vi "init.vi"(8 "error in":errorcluster, 10 "TBM module configuration in":refnum<class "TBM module configuration.lvclass">, 11 "fixed channel runtime in":refnum<class "GPIC ScaleAndLimit runtime.lvclass">) -> (0 "error out":errorcluster, 1 "data allocations":T1, 2 "execution settings":T4, 3 "fixed channel runtime out":refnum<class "GPIC ScaleAndLimit runtime.lvclass">)   [LabVIEW 2015, in "GPIC ScaleAndLimit runtime.lvclass"]
doc: "Provides an interface for initializing a module at runtime. While this interface performs no operations, a child should provide an override which may open any necessary references or sessions, allocate necessary memory, and perform any final configuration validataion before providing the full configuration <b>execution data</b> to the calling process."
uses:
  GPIC ScaleAndLimit runtime.lvclass
  <vilib>/NI/Tag Bus Module Framework/module configuration/TBM module configuration.lvclass
  <vilib>/NI/Tag Bus Module Framework/runtime/execution settings.ctl
  <vilib>/NI/Tag Bus Module Framework/channel/data tables.ctl
  <vilib>/NI/Tag Bus/dictionary/data dictionary.lvclass
  <vilib>/NI/Tag Bus/dictionary table pair.ctl
  <vilib>/NI/Tag Bus/table/data table.ctl
  <vilib>/NI/Tag Bus Module Framework/FPGA manager/methods.ctl
  <vilib>/userdefined/High Color/nirio_resource_hc.ctl
  Interface/FPGAInterface.ctl
  configuration/GPIC ScaleAndLimit configuration.lvclass
  Interface/Configuration.ctl
  GPIC ScaleAndLimit runtime.lvclass/GPIC ScaleAndLimit runtime.ctl
  <vilib>/NI/DCAF/Tag Editor Core/control module/runtime/control module runtime.lvclass
  <vilib>/NI/Tag Bus Module Framework/FPGA manager/FPGA manager.lvlib
  Interface/ScaleAndLimitInterface.lvlib
  <vilib>/NI/Tag Bus Module Framework/runtime/TBM module execution interface.lvclass
  <vilib>/NI/Tag Bus Module Framework/channel/TBM channel.lvclass
  <vilib>/NI/Tag Bus/tag bus.lvlib
  <vilib>/NI/Tag Bus/table/data table.lvlib
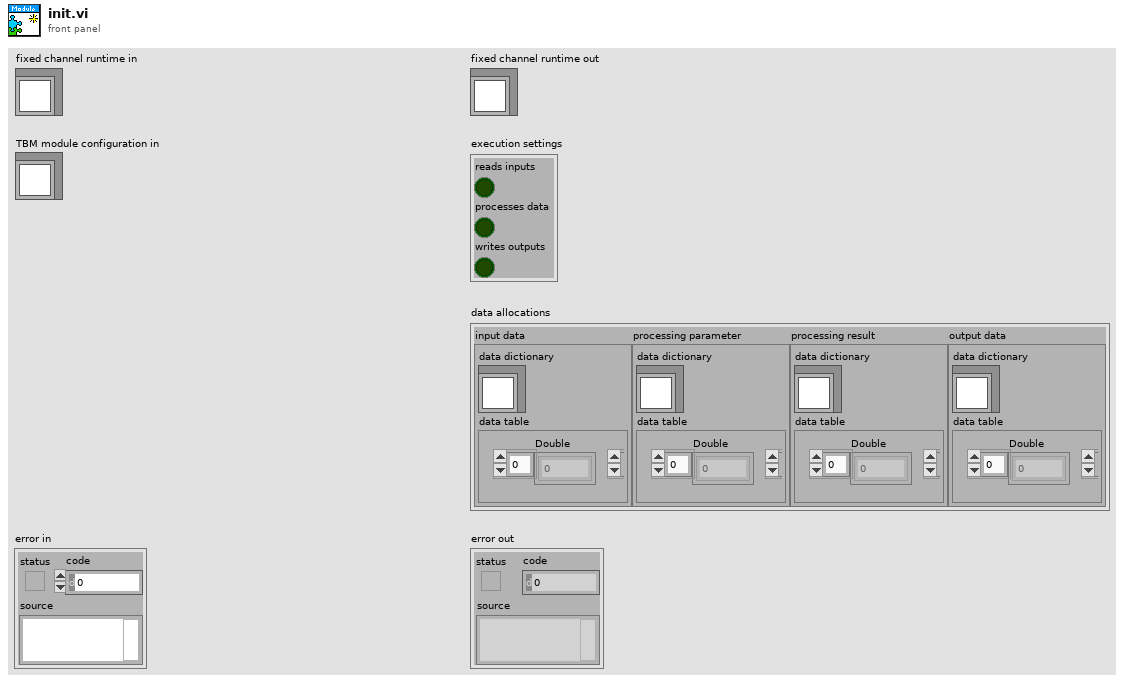
[diagram p1: front panel]
types:
  T1 = typedef "TBM channel.lvclass/data tables.ctl" = cluster{"input data":T2, "processing parameter":T2, "processing result":T2, "output data":T2}
  T2 = typedef "tag bus.lvlib/dictionary table pair.ctl" = cluster{"data dictionary":refnum<class "data dictionary.lvclass">, "data table":T3}
  T3 = typedef "tag bus.lvlib/data table.lvlib/data table.ctl" = cluster{"Double":dbl[], "Single":sgl[], "I64":i64[], "I32":i32[], "I16":i16[], "I8":i8[], "U64":u64[], "U32":u32[], "U16":u16[], "U8":u8[], "Boolean":bool[], "String":string[], "Array of Double":cluster{"DBL Array":dbl[]}[], "Array of Single":cluster{"SGL Array":sgl[]}[], "Array of I64":cluster{"I64 Array":i64[]}[], "Array of I32":cluster{"I32 Array":i32[]}[], "Array of I16":cluster{"I16 Array":i16[]}[], "Array of I8":cluster{"I8 Array":i8[]}[], "Array of U64":cluster{"U64 Array":u64[]}[], "Array of U32":cluster{"U32 Array":u32[]}[], "Array of U16":cluster{"U16 Array":u16[]}[], "Array of U8":cluster{"U8 Array":u8[]}[], "Array of Boolean":cluster{"Boolean Array":bool[]}[], "Array of String":cluster{"String Array":string[]}[]}
  T4 = typedef "TBM module execution interface.lvclass/execution settings.ctl" = cluster{"reads inputs":bool, "processes data":bool, "writes outputs":bool}
  T5 = typedef "ScaleAndLimitInterface.lvlib/Configuration.ctl" = cluster{"Name":string, "M":dbl, "B":i16, "HighLimit":dbl, "LowLimit":dbl, "LimitsEnabled":bool}
  T6 = typedef "ScaleAndLimitInterface.lvlib/FPGAInterface.ctl" = refnum<k20>
  T7 = typedef "nirio_resource_hc.ctl" = tag
  T8 = typedef "FPGA manager.lvlib/methods.ctl" = enum16{"initialize bitfile", "cache bitfile", "locate bitfile", "close bitfile", "clear manager"}
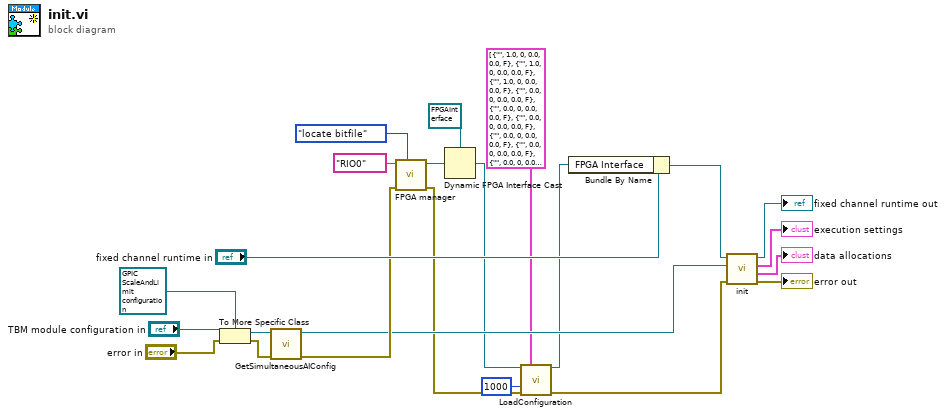
[diagram p0: block diagram]
diagram:
  n1 = To More Specific Class(target class=refnum<class "GPIC ScaleAndLimit configuration.lvclass"> refnum ("GPIC ScaleAndLimit configuration"), reference="TBM module configuration in", error in="error in") -> (specific class reference=w10:refnum<class "GPIC ScaleAndLimit configuration.lvclass">, error out=w9:errorcluster)
  n2 = call "GetSimultaneousAIConfig.vi"("error in (no error)"=w9, "GPIC ScaleAndLimit configuration in"=w10) -> ("error out"=w8:errorcluster, "GPIC ScaleAndLimit configuration out"=w7:refnum<class "GPIC ScaleAndLimit configuration.lvclass">)  [unwired: 7 in, 1 out]
  n3 = call <vilib>:"FPGA manager.vi"("action"=methods."locate bitfile", "error in"=w8, "RIO resource"=T7 "RIO0") -> ("error out"=w5:errorcluster, "bitfile"=w19:refnum<k20>)  [unwired: 6 in, 1 out]
  n4 = Dynamic FPGA Interface Cast(Session In=T6 refnum ("FPGA Interface"), Type=w19) -> (Session Out=w6:T6)
  n5 = call "LoadConfiguration.vi"("FPGA Interface in"=w6, "Configuration"=T5[] [{"Name"="", "M"=1.0, "B"=0, "HighLimit"=0.0, "LowLimit"=0.0, "LimitsEnabled"=FALSE}, {"Name"="", "M"=1.0, "B"=0, "HighLimit"=0.0, "LowLimit"=0.0, "LimitsEnabled"=FALSE}, {"Name"="", "M"=1.0, "B"=0, "HighLimit"=0.0, "LowLimit"=0.0, "LimitsEnabled"=FALSE}, {"Name"="", "M"=0.0, "B"=0, "HighLimit"=0.0, "LowLimit"=0.0, "LimitsEnabled"=FALSE}, {"Name"="", "M"=0.0, "B"=0, "HighLimit"=0.0, "LowLimit"=0.0, "LimitsEnabled"=FALSE}, {"Name"="", "M"=0.0, "B"=0, "HighLimit"=0.0, "LowLimit"=0.0, "LimitsEnabled"=FALSE}, {"Name"="", "M"=0.0, "B"=0, "HighLimit"=0.0, "LowLimit"=0.0, "LimitsEnabled"=FALSE}, {"Name"="", "M"=0.0, "B"=0, "HighLimit"=0.0, "LowLimit"=0.0, "LimitsEnabled"=FALSE}, {"Name"="", "M"=0.0, "B"=0, "HighLimit"=0.0, "LowLimit"=0.0, "LimitsEnabled"=FALSE}, {"Name"="", "M"=0.0, "B"=0, "HighLimit"=0.0, "LowLimit"=0.0, "LimitsEnabled"=FALSE}, {"Name"="", "M"=0.0, "B"=0, "HighLimit"=0.0, "LowLimit"=0.0, "LimitsEnabled"=FALSE}, {"Name"="", "M"=0.0, "B"=0, "HighLimit"=0.0, "LowLimit"=0.0, "LimitsEnabled"=FALSE}, {"Name"="", "M"=0.0, "B"=0, "HighLimit"=0.0, "LowLimit"=0.0, "LimitsEnabled"=FALSE}, {"Name"="", "M"=0.0, "B"=0, "HighLimit"=0.0, "LowLimit"=0.0, "LimitsEnabled"=FALSE}, {"Name"="", "M"=0.0, "B"=0, "HighLimit"=0.0, "LowLimit"=0.0, "LimitsEnabled"=FALSE}, {"Name"="", "M"=1.0, "B"=0, "HighLimit"=0.0, "LowLimit"=0.0, "LimitsEnabled"=FALSE}], "Timeout (ms)"=1000, "error in (no error)"=w5) -> ("FPGA Interface out"=w2:T6, "error out"=w3:errorcluster)  [unwired: 10 in]
  n6 = Bundle By Name(cluster="fixed channel runtime in", "FPGA Interface"=w2) -> (w14:refnum<class "GPIC ScaleAndLimit runtime.lvclass">)
  n7 = call-parent "init.vi"("error in"=w3, "TBM module configuration in"=w7, "fixed channel runtime in"=w14) -> ("error out"=→"error out":errorcluster, "data allocations"=→"data allocations":T1, "execution settings"=→"execution settings":T4, "fixed channel runtime out"=→"fixed channel runtime out":refnum<class "GPIC ScaleAndLimit runtime.lvclass">)  [unwired: 5 in]
